vi "pp2_updateStateInfoState.vi"(10 "New state exit ms increment":i32 min=0, 11 "State In":T2={"Curr  tr"=0, "Curr (ms)"=0, "Cum (ms)"=0, "Run loop diff"=0, "Exit (ms)"=0, "Curr State"=enum."0 Initialization", "Prev State"=enum."0 Initialization", "Side"=FALSE, "Sw1"=FALSE, "Tone Gate"=FALSE, "Stim"=FALSE, "Sw2"=FALSE, "Curr code"=0, "Current Trial"={"Trial Type Number"=1, "Trial Type"=enum."GO", "Trial Weight"=100, "Shock (mA)"=0.3, "Duration (ms)"=0.25, "Type"=enum."04 FM Sweep", "Stim P2"=4000.0, "Stim P3"=0.0, "Stim P4"=0.0, "Stim P1"=2000.0}, "Last tone"=0, "Countdown (s)"=0} {"Current Trial"."Shock (mA)" min=-1.0 max=5.0; "Current Trial"."Trial Weight" step=1; "Current Trial"."Duration (ms)" min=0.0 max=1.0; "Current Trial"."Trial Type Number" min=1 max=256 step=1; "Curr code" format="%b"}) -> (3 "State Out":T2={"Curr  tr"=0, "Curr (ms)"=0, "Cum (ms)"=0, "Run loop diff"=0, "Exit (ms)"=0, "Curr State"=enum."0 Initialization", "Prev State"=enum."0 Initialization", "Side"=FALSE, "Sw1"=FALSE, "Tone Gate"=FALSE, "Stim"=FALSE, "Sw2"=FALSE, "Curr code"=0, "Current Trial"={"Trial Type Number"=1, "Trial Type"=enum."GO", "Trial Weight"=100, "Shock (mA)"=0.3, "Duration (ms)"=0.25, "Type"=enum."04 FM Sweep", "Stim P2"=4000.0, "Stim P3"=0.0, "Stim P4"=0.0, "Stim P1"=2000.0}, "Last tone"=0, "Countdown (s)"=0} {"Current Trial"."Shock (mA)" min=-1.0 max=5.0; "Current Trial"."Trial Weight" step=1; "Current Trial"."Duration (ms)" min=0.0 max=1.0; "Current Trial"."Trial Type Number" min=1 max=256 step=1; "Curr code" format="%b"})   [LabVIEW 2013]
uses:
  pp2_State.ctl
  pp2_CTL_StateInfo.ctl
  pp2_TrialType.ctl
  labolabo2/waveforms/WFTypes.ctl
  pp2_Trial.ctl
panel:
  in  "New State":T1=enum."1 Habituation"
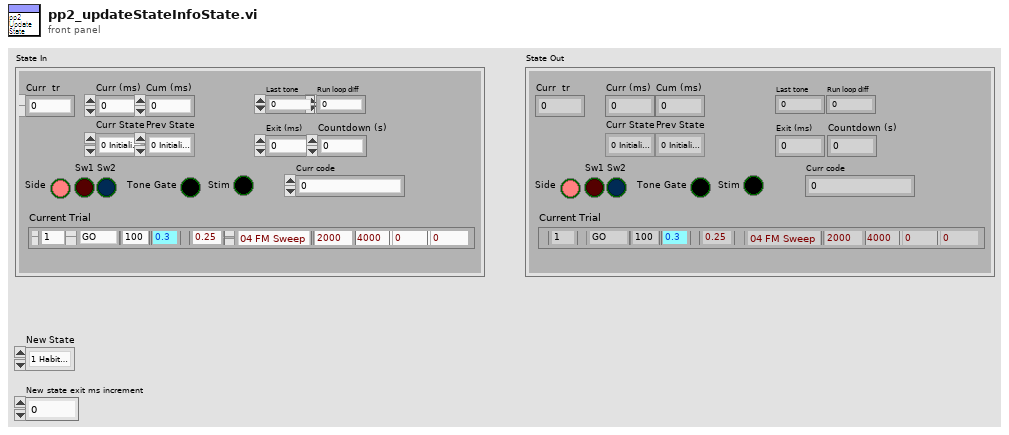
[diagram p1: front panel]
types:
  T1 = typedef "pp2_State.ctl" = enum8{"0 Initialization", "1 Habituation", "2 Load next", "3 Wait", "4 GO Trial", "5 GO Jumped", "6 GO Timeout", "7 NOGO Trial", "8 NOGO Jumped", "9 NOGO Timeout", "10 TEST Trial", "11 TEST Jumped", "12 TEST Timeout", "13 Done"}
  T2 = typedef "pp2_CTL_StateInfo.ctl" = cluster{"Curr  tr":u16, "Curr (ms)":i64, "Cum (ms)":i64, "Run loop diff":i64, "Exit (ms)":i64, "Curr State":T1, "Prev State":T1, "Side":bool, "Sw1":bool, "Tone Gate":bool, "Stim":bool, "Sw2":bool, "Curr code":u8, "Current Trial":T3, "Last tone":i64, "Countdown (s)":i64}
  T3 = typedef "pp2_Trial.ctl" = cluster{"Trial Type Number":i16, "Trial Type":T4, "Trial Weight":u32, "Shock (mA)":dbl, "Duration (ms)":dbl, "Type":T5, "Stim P2":dbl, "Stim P3":dbl, "Stim P4":dbl, "Stim P1":dbl}
  T4 = typedef "pp2_TrialType.ctl" = enum16{"OFF", "GO", "NOGO", "TEST"}
  T5 = typedef "WFTypes.ctl" = enum16{"00 NULL", "01 DC", "02 Noise", "03 Pure Tone", "04 FM Sweep"}
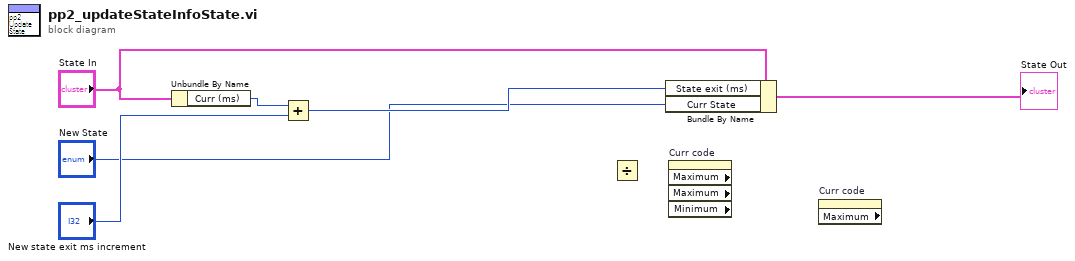
[diagram p0: block diagram]
diagram:
  n1 = Unbundle By Name("State In") -> ("Curr (ms)"=w4:i64)
  n2 = Add(x=w4, y="New state exit ms increment") -> (x+y=w3:i64)
  n3 = Divide() -> ()  [unwired: 2 in, 1 out]
  n4 = Bundle By Name(cluster="State In", "State exit (ms)"=w3, "Curr State"="New State") -> (→"State Out":T2)
  n5 = property on="Curr code" class="DigNum (strict)" props=["Maximum", "Maximum", "Minimum"]() -> ()  [unwired: 2 in, 5 out]
  n6 = property on="Curr code" class="DigNum (strict)" props=["Maximum"]() -> ()  [unwired: 2 in, 3 out]
